vi "PPMSDR - lockin_Vsg_multichannel.vi"(6 "Vmax (end)":dbl=0.00436 format="%#_3p", 8 "Vmin (start)":dbl=-0.00364 format="%#_3p", 9 "Channels: AO":T1={"AO amp (V)"=[0.0001, 0.0, 0.0, 0.0], "AO DC (V)"=[0.00031, -0.00376, 0.0, 0.004], "AO f (Hz)"=[9.468, 0.0, 0.0, 0.0], "AO phi (deg)"=[0.0, 0.0, 0.0, 0.0], "function"=[enum."Sine Wave", enum."Sine Wave", enum."Sine Wave", enum."Sine Wave"]} {"AO DC (V)" format="%#_6p"; "AO amp (V)" format="%#_6p"}, 10 "Comments":string="DC sweep from -3.69mV to 4.31mV, 5uV step\nDragPotential sweep from -4mV to 4mV, 400uV step\nB = 0T\nT = 218mK\nVbg = 0V\nTC = 0.1s\n\nI+/-: 2/5 100uVac + DC sweep, 9.468Hz\nI2+: 28  0Vac + value according to dragpotential sweep(offset 240uV), 0Hz\nI2-: 3 0Vac + DragPotential sweep, 0Hz\nV+/-: 1/4\nV2+/-: 28/27\nV3+/-: 28/3\nappliedPotential= 0.004000", 11 "ITX folder":string="15-DragPotentialsweep-I-LDr25-RGND-Lockin") -> ()   [LabVIEW 2013]
uses:
  <userlib>/Levylab/PPMS VI/SubVI/ITX_Global.vi
  QDServer/QDServGlobal.vi
  Labview_Local/Lockin-4461_Multiple Inputs and Outputs_KH Folder/P/users1/Joe/Lockin-4461_3.0 4461-4462 Multichannel Folder/DAQ-Lockin-SubVI/Lock-in Globles Multiple Inputs and Outputs.vi
  cryogenic ltd/state machine/state machine/Cryogeni Global 1.vi
panel:
  in  "dV 2":dbl=0.0002 format="%#_3p"
  in  "Vend":dbl=-5.0 format="%#_3p"
  in  "Vstart":dbl=-4.8 format="%#_3p"
  in  "Tab Control":enum32{"Sweep BG", "lockin/SG Control", "Data"}(tab)=enum."lockin/SG Control"
  in  "dV":dbl=5e-06 format="%#_3p"
  out "T (mK)":dbl=0.24
  in  "wait between Vsgs":u32=50
  in  "Initial wait":u32=6000
  in  "# of lockins * #freq":i32=10
  in  "\"channel\" side gate":i32
  in  "T=sg\nF=bg":bool=TRUE
  in  "cycles (1,2,...)":i32=1 min=1 step=1
  in  "phase":dbl
  out "ramp rate":dbl=0.0214 format="%#_13g"
  out "Field":dbl=0.051 format="%#_13g"
  in  "function (ramp)":enum16{"Ramp", "Triangle", "Sine"}(ring)
  in  "Expt?":bool=TRUE
  out "Waveform Graph":dbl[](graph)=[-0.0036900000000000006, -0.0036850000000000008, -0.0036800000000000005, -0.0036750000000000007, -0.0036700000000000005, -0.0036650000000000007, -0.0036600000000000005, -0.0036550000000000007, -0.0036500000000000005, -0.0036450000000000007, -0.0036400000000000004, -0.0036350000000000006, -0.0036300000000000004, -0.0036250000000000006, -0.0036200000000000004, -0.0036150000000000006, -0.0036100000000000004, -0.0036050000000000006, -0.0036000000000000008, -0.0035950000000000005, -0.0035900000000000007, -0.0035850000000000005, -0.0035800000000000007, -0.0035750000000000005, -0.0035700000000000007, -0.0035650000000000005, -0.0035600000000000007, -0.0035550000000000004, -0.0035500000000000006, -0.0035450000000000004, -0.0035400000000000006, -0.0035350000000000004, -0.0035300000000000006, -0.0035250000000000004, -0.0035200000000000006, -0.0035150000000000008, -0.0035100000000000005, -0.0035050000000000007, -0.0035000000000000005, -0.0034950000000000007, -0.0034900000000000005, -0.0034850000000000007, -0.0034800000000000005, -0.0034750000000000007, -0.0034700000000000004, -0.0034650000000000006, -0.0034600000000000004, -0.0034550000000000006, -0.0034500000000000004, -0.0034450000000000006, -0.0034400000000000003, -0.0034350000000000006, -0.0034300000000000008, -0.0034250000000000005, -0.0034200000000000007, -0.0034150000000000005, -0.0034100000000000007, -0.0034050000000000005, -0.0034000000000000007, -0.0033950000000000004, -0.0033900000000000007, -0.0033850000000000004, -0.0033800000000000006, -0.0033750000000000004, -0.0033700000000000006, -0.0033650000000000004, -0.0033600000000000006, -0.0033550000000000003, -0.0033500000000000005, -0.0033450000000000008, -0.0033400000000000005, -0.0033350000000000007, -0.0033300000000000005, -0.0033250000000000007, -0.0033200000000000005, -0.0033150000000000007, -0.0033100000000000004, -0.0033050000000000006, -0.0033000000000000004, -0.0032950000000000006, -0.0032900000000000004, -0.0032850000000000006, -0.0032800000000000004, -0.0032750000000000006, -0.0032700000000000003, -0.0032650000000000005, -0.0032600000000000007, -0.0032550000000000005, -0.0032500000000000007, -0.0032450000000000005, -0.0032400000000000007, -0.0032350000000000005, -0.0032300000000000007, -0.0032250000000000004, -0.0032200000000000006, -0.0032150000000000004, -0.0032100000000000006, -0.0032050000000000004, -0.0032000000000000006, -0.003195000000000001, -0.0031900000000000006, -0.0031850000000000003, -0.0031800000000000005, -0.0031750000000000007, -0.0031700000000000005, -0.0031650000000000003, -0.0031600000000000005, -0.0031550000000000007, -0.0031500000000000005, -0.0031450000000000007, -0.0031400000000000004, -0.0031350000000000006, -0.0031300000000000004, -0.0031250000000000006, -0.0031200000000000004, -0.0031150000000000006, -0.003110000000000001, -0.0031050000000000006, -0.0031000000000000003, -0.0030950000000000005, -0.0030900000000000007, -0.0030850000000000005, -0.0030800000000000003, -0.0030750000000000005, -0.0030700000000000007, -0.0030650000000000004, -0.0030600000000000007, -0.0030550000000000004, -0.0030500000000000006, -0.0030450000000000004, -0.0030400000000000006, -0.0030350000000000004, -0.0030300000000000006, -0.0030250000000000008, -0.0030200000000000005, -0.0030150000000000003, -0.0030100000000000005, -0.0030050000000000007, -0.0030000000000000005, -0.0029950000000000003, -0.0029900000000000005, -0.0029850000000000007, -0.0029800000000000004, -0.0029750000000000006, -0.0029700000000000004, -0.0029650000000000006, -0.0029600000000000004, -0.0029550000000000006, -0.0029500000000000004, -0.0029450000000000006, -0.0029400000000000008, -0.0029350000000000005, -0.0029300000000000003, -0.0029250000000000005, -0.0029200000000000007, -0.0029150000000000005, -0.0029100000000000003, -0.0029050000000000005, -0.0029000000000000007, -0.0028950000000000004, -0.0028900000000000006, -0.0028850000000000004, -0.0028800000000000006, -0.0028750000000000004, -0.0028700000000000006, -0.0028650000000000004, -0.0028600000000000006, -0.0028550000000000008, -0.0028500000000000005, -0.0028450000000000003, -0.0028400000000000005, -0.0028350000000000007, -0.0028300000000000005, -0.0028250000000000003, -0.0028200000000000005, -0.0028150000000000007, -0.0028100000000000004, -0.0028050000000000006, -0.0028000000000000004, -0.0027950000000000006, -0.0027900000000000004, -0.0027850000000000006, -0.0027800000000000004, -0.0027750000000000006, -0.0027700000000000008, -0.0027650000000000005, -0.0027600000000000003, -0.0027550000000000005, -0.0027500000000000007, -0.0027450000000000005, -0.0027400000000000002, -0.0027350000000000005, -0.0027300000000000007, -0.0027250000000000004, -0.0027200000000000006, -0.0027150000000000004, -0.0027100000000000006, -0.002705000000000001, -0.0027000000000000006, -0.0026950000000000003, -0.0026900000000000006, -0.0026850000000000008, -0.0026800000000000005, -0.0026750000000000003, -0.0026700000000000005, -0.0026650000000000007, -0.0026600000000000005, -0.0026550000000000002, -0.0026500000000000004, -0.0026450000000000006, -0.0026400000000000004, -0.002635, -0.0026300000000000004, -0.0026250000000000006, -0.002620000000000001, -0.0026150000000000006, -0.0026100000000000003, -0.0026050000000000005, -0.0026000000000000007, -0.0025950000000000005, -0.0025900000000000003, -0.0025850000000000005, -0.0025800000000000007, -0.0025750000000000005, -0.0025700000000000002, -0.0025650000000000004, -0.0025600000000000006, -0.0025550000000000004, -0.00255, -0.0025450000000000004, -0.0025400000000000006, -0.002535000000000001, -0.0025300000000000006, -0.0025250000000000003, -0.0025200000000000005, -0.0025150000000000007, -0.0025100000000000005, -0.0025050000000000003, -0.0025000000000000005, -0.0024950000000000007, -0.0024900000000000005, -0.0024850000000000002, -0.0024800000000000004, -0.0024750000000000006, -0.0024700000000000004, -0.002465, -0.0024600000000000004, -0.0024550000000000006, -0.002450000000000001, -0.0024450000000000006, -0.0024400000000000003, -0.0024350000000000005, -0.0024300000000000007, -0.0024250000000000005, -0.0024200000000000003, -0.0024150000000000005, -0.0024100000000000007, -0.0024050000000000005, -0.0024000000000000002, -0.0023950000000000004, -0.0023900000000000006, -0.0023850000000000004, -0.00238, -0.0023750000000000004, -0.0023700000000000006, -0.0023650000000000008, -0.0023600000000000006, -0.0023550000000000003, -0.0023500000000000005, -0.0023450000000000007, -0.0023400000000000005, -0.0023350000000000003, -0.0023300000000000005, -0.0023250000000000007, -0.0023200000000000004, -0.0023150000000000002, -0.0023100000000000004, -0.0023050000000000006, -0.0023000000000000004, -0.002295, -0.0022900000000000004, -0.0022850000000000006, -0.0022800000000000008, -0.0022750000000000005, -0.0022700000000000003, -0.0022650000000000005, -0.0022600000000000007, -0.0022550000000000005, -0.0022500000000000003, -0.0022450000000000005, -0.0022400000000000007, -0.0022350000000000004, -0.00223, -0.0022250000000000004, -0.0022200000000000006, -0.0022150000000000004, -0.00221, -0.0022050000000000004, -0.0022000000000000006, -0.0021950000000000008, -0.0021900000000000005, -0.0021850000000000003, -0.0021800000000000005, -0.0021750000000000007, -0.0021700000000000005, -0.0021650000000000003, -0.0021600000000000005, -0.0021550000000000007, -0.0021500000000000004, -0.002145, -0.0021400000000000004, -0.0021350000000000006, -0.0021300000000000004, -0.002125, -0.0021200000000000004, -0.0021150000000000006, -0.0021100000000000008, -0.0021050000000000005, -0.0021000000000000003, -0.0020950000000000005, -0.0020900000000000007, -0.0020850000000000005, -0.0020800000000000003, -0.0020750000000000005, -0.0020700000000000007, -0.0020650000000000004, -0.00206, -0.0020550000000000004, -0.0020500000000000006, -0.0020450000000000004, -0.00204, -0.0020350000000000004, -0.0020300000000000006, -0.0020250000000000008, -0.0020200000000000005, -0.0020150000000000003, -0.0020100000000000005, -0.0020050000000000007, -0.0020000000000000005, -0.0019950000000000002, -0.0019900000000000004, -0.0019850000000000007, -0.0019800000000000004, -0.001975, -0.0019700000000000004, -0.0019650000000000006, -0.0019600000000000004, -0.001955, -0.0019500000000000003, -0.0019450000000000003, -0.0019400000000000005, -0.0019350000000000005, -0.0019300000000000005, -0.0019250000000000005, -0.0019200000000000005, -0.0019150000000000005, -0.0019100000000000005, -0.0019050000000000004, -0.0019000000000000004, -0.0018950000000000004, -0.0018900000000000004, -0.0018850000000000004, -0.0018800000000000004, -0.0018750000000000004, -0.0018700000000000004, -0.0018650000000000003, -0.0018600000000000003, -0.0018550000000000005, -0.0018500000000000005, -0.0018450000000000005, -0.0018400000000000005, -0.0018350000000000005, -0.0018300000000000005, -0.0018250000000000004, -0.0018200000000000004, -0.0018150000000000004, -0.0018100000000000004, -0.0018050000000000004, -0.0018000000000000004, -0.0017950000000000004, -0.0017900000000000004, -0.0017850000000000003, -0.0017800000000000003, -0.0017750000000000003, -0.0017700000000000003, -0.0017650000000000005, -0.0017600000000000005, -0.0017550000000000005, -0.0017500000000000005, -0.0017450000000000005, -0.0017400000000000004, -0.0017350000000000004, -0.0017300000000000002, -0.0017250000000000004, -0.0017200000000000006, -0.0017150000000000004, -0.0017100000000000006, -0.0017050000000000004, -0.0017000000000000006, -0.0016950000000000003, -0.0016900000000000005, -0.0016850000000000003, -0.0016800000000000005, -0.0016750000000000003, -0.0016700000000000005, -0.0016650000000000002, -0.0016600000000000005, -0.0016550000000000002, -0.0016500000000000004, -0.0016450000000000002, -0.0016400000000000004, -0.0016350000000000006, -0.0016300000000000004, -0.0016250000000000006, -0.0016200000000000003, -0.0016150000000000005, -0.0016100000000000003, -0.0016050000000000005, -0.0016000000000000003, -0.0015950000000000005, -0.0015900000000000003, -0.0015850000000000005, -0.0015800000000000002, -0.0015750000000000004, -0.0015700000000000002, -0.0015650000000000004, -0.0015600000000000002, -0.0015550000000000004, -0.0015500000000000006, -0.0015450000000000004, -0.0015400000000000006, -0.0015350000000000003, -0.0015300000000000005, -0.0015250000000000003, -0.0015200000000000005, -0.0015150000000000003, -0.0015100000000000005, -0.0015050000000000003, -0.0015000000000000005, -0.0014950000000000002, -0.0014900000000000004, -0.0014850000000000002, -0.0014800000000000004, -0.0014750000000000002, -0.0014700000000000004, -0.0014650000000000006, -0.0014600000000000004, -0.0014550000000000006, -0.0014500000000000003, -0.0014450000000000005, -0.0014400000000000003, -0.0014350000000000005, -0.0014300000000000003, -0.0014250000000000005, -0.0014200000000000003, -0.0014150000000000005, -0.0014100000000000002, -0.0014050000000000004, -0.0014000000000000002, -0.0013950000000000004, -0.0013900000000000002, -0.0013850000000000004, -0.0013800000000000006, -0.0013750000000000004, -0.0013700000000000006, -0.0013650000000000003, -0.0013600000000000005, -0.0013550000000000003, -0.0013500000000000005, -0.0013450000000000003, -0.0013400000000000005, -0.0013350000000000002, -0.0013300000000000005, -0.0013250000000000002, -0.0013200000000000004, -0.0013150000000000002, -0.0013100000000000004, -0.0013050000000000002, -0.0013000000000000004, -0.0012950000000000006, -0.0012900000000000003, -0.0012850000000000006, -0.0012800000000000003, -0.0012750000000000005, -0.0012700000000000003, -0.0012650000000000005, -0.0012600000000000003, -0.0012550000000000005, -0.0012500000000000002, -0.0012450000000000004, -0.0012400000000000002, -0.0012350000000000004, -0.0012300000000000002, -0.0012250000000000004, -0.0012200000000000002, -0.0012150000000000004, -0.0012100000000000006, -0.0012050000000000003, -0.0012000000000000005, -0.0011950000000000003, -0.0011900000000000005, -0.0011850000000000003, -0.0011800000000000005, -0.0011750000000000003, -0.0011700000000000005, -0.0011650000000000002, -0.0011600000000000004, -0.0011550000000000002, -0.0011500000000000004, -0.0011450000000000002, -0.0011400000000000004, -0.0011350000000000002, -0.0011300000000000004, -0.0011250000000000006, -0.0011200000000000003, -0.0011150000000000005, -0.0011100000000000003, -0.0011050000000000005, -0.0011000000000000003, -0.0010950000000000005, -0.0010900000000000003, -0.0010850000000000005, -0.0010800000000000002, -0.0010750000000000004, -0.0010700000000000002, -0.0010650000000000004, -0.0010600000000000002, -0.0010550000000000004, -0.0010500000000000002, -0.0010450000000000004, -0.0010400000000000006, -0.0010350000000000003, -0.0010300000000000005, -0.0010250000000000003, -0.0010200000000000005, -0.0010150000000000003, -0.0010100000000000005, -0.0010050000000000003, -0.0010000000000000005, -0.0009950000000000002, -0.0009900000000000004, -0.0009850000000000002, -0.0009800000000000004, -0.0009750000000000002, -0.0009700000000000004, -0.0009650000000000001, -0.0009600000000000003, -0.0009550000000000006, -0.0009500000000000003, -0.0009450000000000005, -0.0009400000000000003, -0.0009350000000000005, -0.0009300000000000003, -0.0009250000000000005, -0.0009200000000000002, -0.0009150000000000004, -0.0009100000000000002, -0.0009050000000000004, -0.0009000000000000002, -0.0008950000000000004, -0.0008900000000000002, -0.0008850000000000004, -0.0008800000000000001, -0.0008750000000000003, -0.0008700000000000005, -0.0008650000000000003, -0.0008600000000000005, -0.0008550000000000003, -0.0008500000000000005, -0.0008450000000000003, -0.0008400000000000005, -0.0008350000000000002, -0.0008300000000000004, -0.0008250000000000002, -0.0008200000000000004, -0.0008150000000000002, -0.0008100000000000004, -0.0008050000000000002, -0.0008000000000000004, -0.0007950000000000001, -0.0007900000000000003, -0.0007850000000000005, -0.0007800000000000003, -0.0007750000000000005, -0.0007700000000000003, -0.0007650000000000005, -0.0007600000000000003, -0.0007550000000000005, -0.0007500000000000002, -0.0007450000000000004, -0.0007400000000000002, -0.0007350000000000004, -0.0007300000000000002, -0.0007250000000000004, -0.0007200000000000002, -0.0007150000000000004, -0.0007100000000000001, -0.0007050000000000003, -0.0007000000000000005, -0.0006950000000000003, -0.0006900000000000005, -0.0006850000000000003, -0.0006800000000000005, -0.0006750000000000003, -0.0006700000000000005, -0.0006650000000000002, -0.0006600000000000004, -0.0006550000000000002, -0.0006500000000000004, -0.0006450000000000002, -0.0006400000000000004, -0.0006350000000000001, -0.0006300000000000004, -0.0006250000000000001, -0.0006200000000000003, -0.0006150000000000005, -0.0006100000000000003, -0.0006050000000000005, -0.0006000000000000003, -0.0005950000000000005, -0.0005900000000000002, -0.0005850000000000005, -0.0005800000000000002, -0.0005750000000000004, -0.0005700000000000002, -0.0005650000000000004, -0.0005600000000000002, -0.0005550000000000004, -0.0005500000000000001, -0.0005450000000000003, -0.0005400000000000001, -0.0005350000000000003, -0.0005300000000000005, -0.0005250000000000003, -0.0005200000000000005, -0.0005150000000000003, -0.0005100000000000005, -0.0005050000000000002, -0.0005000000000000004, -0.0004950000000000002, -0.0004900000000000004, -0.0004850000000000002, -0.0004800000000000004, -0.00047500000000000016, -0.00047000000000000037, -0.00046500000000000014, -0.00046000000000000034, -0.0004550000000000001, -0.0004500000000000003, -0.0004450000000000005, -0.0004400000000000003, -0.0004350000000000005, -0.00043000000000000026, -0.00042500000000000046, -0.00042000000000000023, -0.00041500000000000044, -0.0004100000000000002, -0.0004050000000000004, -0.0004000000000000002, -0.0003950000000000004, -0.00039000000000000016, -0.00038500000000000036, -0.00038000000000000013, -0.00037500000000000033, -0.0003700000000000001, -0.0003650000000000003, -0.0003600000000000005, -0.0003550000000000003, -0.0003500000000000005, -0.00034500000000000025, -0.00034000000000000046, -0.00033500000000000023, -0.00033000000000000043, -0.0003250000000000002, -0.0003200000000000004, -0.0003150000000000002, -0.0003100000000000004, -0.00030500000000000015, -0.00030000000000000035, -0.0002950000000000001, -0.0002900000000000003, -0.0002850000000000001, -0.0002800000000000003, -0.0002750000000000005, -0.0002700000000000003, -0.0002650000000000005, -0.00026000000000000025, -0.00025500000000000045, -0.0002500000000000002, -0.0002450000000000004, -0.0002400000000000002, -0.0002350000000000004, -0.00023000000000000017, -0.00022500000000000037, -0.00022000000000000014, -0.00021500000000000035, -0.00021000000000000012, -0.00020500000000000032, -0.0002000000000000001, -0.0001950000000000003, -0.0001900000000000005, -0.00018500000000000027, -0.00018000000000000047, -0.00017500000000000024, -0.00017000000000000045, -0.00016500000000000022, -0.00016000000000000042, -0.0001550000000000002, -0.0001500000000000004, -0.00014500000000000016, -0.00014000000000000037, -0.00013500000000000014, -0.00013000000000000034, -0.0001250000000000001, -0.00012000000000000031, -0.00011500000000000008, -0.00011000000000000029, -0.00010500000000000049, -0.00010000000000000026, -9.500000000000047e-05, -9.000000000000024e-05, -8.500000000000044e-05, -8.000000000000021e-05, -7.500000000000041e-05, -7.000000000000018e-05, -6.500000000000039e-05, -6.000000000000016e-05, -5.500000000000036e-05, -5.000000000000013e-05, -4.5000000000000335e-05, -4.0000000000000105e-05, -3.500000000000031e-05, -3.000000000000008e-05, -2.5000000000000282e-05, -2.0000000000000486e-05, -1.5000000000000256e-05, -1.000000000000046e-05, -5.00000000000023e-06, -4.336808689942018e-19, 4.999999999999796e-06, 9.999999999999593e-06, 1.4999999999999823e-05, 1.999999999999962e-05, 2.499999999999985e-05, 2.9999999999999645e-05, 3.4999999999999875e-05, 3.999999999999967e-05, 4.49999999999999e-05, 4.99999999999997e-05, 5.499999999999993e-05, 5.9999999999999724e-05, 6.499999999999952e-05, 6.999999999999975e-05, 7.499999999999955e-05, 7.999999999999978e-05, 8.499999999999957e-05, 8.99999999999998e-05, 9.49999999999996e-05, 9.999999999999983e-05, 0.00010499999999999962, 0.00010999999999999985, 0.00011499999999999965, 0.00011999999999999988, 0.00012499999999999968, 0.0001299999999999999, 0.0001349999999999997, 0.00013999999999999993, 0.00014499999999999973, 0.00014999999999999996, 0.00015499999999999976, 0.00015999999999999955, 0.00016499999999999978, 0.00016999999999999958, 0.0001749999999999998, 0.0001799999999999996, 0.00018499999999999983, 0.00018999999999999963, 0.00019499999999999986, 0.00019999999999999966, 0.0002049999999999999, 0.00020999999999999968, 0.0002149999999999999, 0.0002199999999999997, 0.0002249999999999995, 0.00023000000000000017, 0.00023499999999999997, 0.00023999999999999976, 0.00024499999999999956, 0.00024999999999999935, 0.000255, 0.0002599999999999998, 0.0002649999999999996, 0.0002699999999999994, 0.00027500000000000007, 0.00027999999999999987, 0.00028499999999999966, 0.00028999999999999946, 0.0002950000000000001, 0.0002999999999999999, 0.0003049999999999997, 0.0003099999999999995, 0.0003150000000000002, 0.00031999999999999997, 0.00032499999999999977, 0.00032999999999999956, 0.00033499999999999936, 0.00034, 0.0003449999999999998, 0.0003499999999999996, 0.0003549999999999994, 0.0003600000000000001, 0.0003649999999999999, 0.00036999999999999967, 0.00037499999999999947, 0.00038000000000000013, 0.0003849999999999999, 0.0003899999999999997, 0.0003949999999999995, 0.0004000000000000002, 0.000405, 0.0004099999999999998, 0.00041499999999999957, 0.00041999999999999937, 0.00042500000000000003, 0.0004299999999999998, 0.0004349999999999996, 0.0004399999999999994, 0.0004450000000000001, 0.0004499999999999999, 0.0004549999999999997, 0.00045999999999999947, 0.00046500000000000014, 0.00046999999999999993, 0.00047499999999999973, 0.0004799999999999995, 0.0004850000000000002, 0.00049, 0.0004949999999999998, 0.0004999999999999996, 0.0005049999999999994, 0.00051, 0.0005149999999999998, 0.0005199999999999996, 0.0005249999999999994, 0.0005300000000000001, 0.0005349999999999999, 0.0005399999999999997, 0.0005449999999999995, 0.0005500000000000001, 0.0005549999999999999, 0.0005599999999999997, 0.0005649999999999995, 0.0005700000000000002, 0.000575, 0.0005799999999999998, 0.0005849999999999996, 0.0005899999999999994, 0.000595, 0.0005999999999999998, 0.0006049999999999996, 0.0006099999999999994, 0.0006150000000000001, 0.0006199999999999999, 0.0006249999999999997, 0.0006299999999999995, 0.0006350000000000001, 0.0006399999999999999, 0.0006449999999999997, 0.0006499999999999995, 0.0006550000000000002, 0.00066, 0.0006649999999999998, 0.0006699999999999996, 0.0006749999999999994, 0.00068, 0.0006849999999999998, 0.0006899999999999996, 0.0006949999999999994, 0.0007000000000000001, 0.0007049999999999999, 0.0007099999999999997, 0.0007149999999999995, 0.0007200000000000002, 0.000725, 0.0007299999999999997, 0.0007349999999999995, 0.0007400000000000002, 0.000745, 0.0007499999999999998, 0.0007549999999999996, 0.0007599999999999994, 0.0007650000000000001, 0.0007699999999999999, 0.0007749999999999996, 0.0007799999999999994, 0.0007850000000000001, 0.0007899999999999999, 0.0007949999999999997, 0.0007999999999999995, 0.0008050000000000002, 0.00081, 0.0008149999999999998, 0.0008199999999999995, 0.0008250000000000002, 0.00083, 0.0008349999999999998, 0.0008399999999999996, 0.0008449999999999994, 0.0008500000000000001, 0.0008549999999999999, 0.0008599999999999997, 0.0008649999999999994, 0.0008700000000000001, 0.0008749999999999999, 0.0008799999999999997, 0.0008849999999999995, 0.0008900000000000002, 0.000895, 0.0008999999999999998, 0.0009049999999999996, 0.0009100000000000002, 0.000915, 0.0009199999999999998, 0.0009249999999999996, 0.0009299999999999994, 0.0009350000000000001, 0.0009399999999999999, 0.0009449999999999997, 0.0009499999999999995, 0.0009550000000000001, 0.0009599999999999999, 0.0009649999999999997, 0.0009699999999999995, 0.0009750000000000002, 0.00098, 0.0009849999999999998, 0.0009899999999999996, 0.0009950000000000002, 0.001, 0.0010049999999999998, 0.0010099999999999996, 0.0010149999999999994, 0.00102, 0.0010249999999999999, 0.0010299999999999997, 0.0010349999999999995, 0.0010400000000000001, 0.001045, 0.0010499999999999997, 0.0010549999999999995, 0.0010600000000000002, 0.001065, 0.0010699999999999998, 0.0010749999999999996, 0.0010800000000000002, 0.001085, 0.0010899999999999998, 0.0010949999999999996, 0.0010999999999999994, 0.001105, 0.0011099999999999999, 0.0011149999999999997, 0.0011199999999999995, 0.0011250000000000001, 0.00113, 0.0011349999999999997, 0.0011399999999999995, 0.0011450000000000002, 0.00115, 0.0011549999999999998, 0.0011599999999999996, 0.0011650000000000002, 0.00117, 0.0011749999999999998, 0.0011799999999999996, 0.0011849999999999994, 0.00119, 0.0011949999999999999, 0.0011999999999999997, 0.0012049999999999995, 0.0012100000000000001, 0.001215, 0.0012199999999999997, 0.0012249999999999995, 0.0012300000000000002, 0.001235, 0.0012399999999999998, 0.0012449999999999996, 0.0012500000000000002, 0.001255, 0.0012599999999999998, 0.0012649999999999996, 0.0012699999999999994, 0.001275, 0.0012799999999999999, 0.0012849999999999997, 0.0012899999999999995, 0.0012950000000000001, 0.0013, 0.0013049999999999997, 0.0013099999999999995, 0.0013150000000000002, 0.00132, 0.0013249999999999998, 0.0013299999999999996, 0.0013350000000000002, 0.00134, 0.0013449999999999998, 0.0013499999999999996, 0.0013549999999999994, 0.00136, 0.001365, 0.0013699999999999997, 0.0013749999999999995, 0.0013800000000000002, 0.001385, 0.0013899999999999997, 0.0013949999999999995, 0.0014000000000000002, 0.001405, 0.0014099999999999998, 0.0014149999999999996, 0.0014200000000000003, 0.001425, 0.0014299999999999998, 0.0014349999999999996, 0.0014399999999999994, 0.001445, 0.00145, 0.0014549999999999997, 0.0014599999999999995, 0.0014650000000000002, 0.00147, 0.0014749999999999997, 0.0014799999999999995, 0.0014850000000000002, 0.00149, 0.0014949999999999998, 0.0014999999999999996, 0.0015050000000000003, 0.00151, 0.0015149999999999999, 0.0015199999999999997, 0.0015249999999999994, 0.0015300000000000001, 0.001535, 0.0015399999999999997, 0.0015449999999999995, 0.0015500000000000002, 0.001555, 0.0015599999999999998, 0.0015649999999999996, 0.0015700000000000002, 0.001575, 0.0015799999999999998, 0.0015849999999999996, 0.0015900000000000003, 0.001595, 0.0015999999999999999, 0.0016049999999999997, 0.0016099999999999995, 0.0016150000000000001, 0.00162, 0.0016249999999999997, 0.0016299999999999995, 0.0016350000000000002, 0.00164, 0.0016449999999999998, 0.0016499999999999996, 0.0016550000000000002, 0.00166, 0.0016649999999999998, 0.0016699999999999996, 0.0016750000000000003, 0.00168, 0.0016849999999999999, 0.0016899999999999997, 0.0016949999999999995, 0.0017000000000000001, 0.001705, 0.0017099999999999997, 0.0017149999999999995, 0.0017200000000000002, 0.001725, 0.0017299999999999998, 0.0017349999999999996, 0.0017400000000000002, 0.001745, 0.0017499999999999998, 0.0017549999999999996, 0.0017600000000000003, 0.001765, 0.0017699999999999999, 0.0017749999999999997, 0.0017799999999999995, 0.0017850000000000001, 0.00179, 0.0017949999999999997, 0.0017999999999999995, 0.0018050000000000002, 0.00181, 0.0018149999999999998, 0.0018199999999999996, 0.0018250000000000002, 0.00183, 0.0018349999999999998, 0.0018399999999999996, 0.0018450000000000003, 0.00185, 0.0018549999999999999, 0.0018599999999999997, 0.0018649999999999995, 0.0018700000000000001, 0.001875, 0.0018799999999999997, 0.0018849999999999995, 0.0018900000000000002, 0.001895, 0.0018999999999999998, 0.0019049999999999996, 0.0019100000000000002, 0.001915, 0.0019199999999999998, 0.0019249999999999996, 0.0019300000000000003, 0.001935, 0.0019399999999999999, 0.0019449999999999997, 0.0019499999999999995, 0.001955, 0.00196, 0.0019649999999999997, 0.0019699999999999995, 0.001975, 0.00198, 0.001985, 0.0019899999999999996, 0.0019950000000000002, 0.002, 0.002005, 0.0020099999999999996, 0.0020150000000000003, 0.00202, 0.002025, 0.0020299999999999997, 0.0020349999999999995, 0.00204, 0.002045, 0.0020499999999999997, 0.0020549999999999995, 0.00206, 0.002065, 0.00207, 0.0020749999999999996, 0.0020800000000000003, 0.002085, 0.00209, 0.0020949999999999996, 0.0021000000000000003, 0.002105, 0.00211, 0.0021149999999999997, 0.0021199999999999995, 0.002125, 0.00213, 0.0021349999999999997, 0.0021399999999999995, 0.002145, 0.00215, 0.002155, 0.0021599999999999996, 0.0021650000000000003, 0.00217, 0.002175, 0.0021799999999999996, 0.0021850000000000003, 0.00219, 0.002195, 0.0021999999999999997, 0.0022049999999999995, 0.00221, 0.002215, 0.0022199999999999998, 0.0022249999999999995, 0.00223, 0.002235, 0.00224, 0.0022449999999999996, 0.0022500000000000003, 0.002255, 0.00226, 0.0022649999999999997, 0.0022700000000000003, 0.002275, 0.00228, 0.0022849999999999997, 0.0022899999999999995, 0.002295, 0.0023, 0.0023049999999999998, 0.0023099999999999996, 0.0023150000000000002, 0.00232, 0.002325, 0.0023299999999999996, 0.0023350000000000003, 0.00234, 0.002345, 0.0023499999999999997, 0.0023550000000000003, 0.00236, 0.002365, 0.0023699999999999997, 0.0023749999999999995, 0.00238, 0.002385, 0.0023899999999999998, 0.0023949999999999996, 0.0024000000000000002, 0.002405, 0.00241, 0.0024149999999999996, 0.0024200000000000003, 0.002425, 0.00243, 0.0024349999999999997, 0.0024400000000000003, 0.002445, 0.00245, 0.0024549999999999997, 0.0024599999999999995, 0.002465, 0.00247, 0.0024749999999999998, 0.0024799999999999996, 0.0024850000000000002, 0.00249, 0.002495, 0.0024999999999999996, 0.0025050000000000003, 0.00251, 0.002515, 0.0025199999999999997, 0.0025250000000000003, 0.00253, 0.002535, 0.0025399999999999997, 0.0025449999999999995, 0.00255, 0.002555, 0.0025599999999999998, 0.0025649999999999996, 0.0025700000000000002, 0.002575, 0.00258, 0.0025849999999999996, 0.0025900000000000003, 0.002595, 0.0026, 0.0026049999999999997, 0.0026100000000000003, 0.002615, 0.00262, 0.0026249999999999997, 0.0026299999999999995, 0.002635, 0.00264, 0.0026449999999999998, 0.0026499999999999996, 0.0026550000000000002, 0.00266, 0.002665, 0.0026699999999999996, 0.0026750000000000003, 0.00268, 0.002685, 0.0026899999999999997, 0.0026950000000000003, 0.0027, 0.002705, 0.0027099999999999997, 0.0027149999999999995, 0.00272, 0.002725, 0.00273, 0.0027349999999999996, 0.0027400000000000002, 0.002745, 0.00275, 0.0027549999999999996, 0.0027600000000000003, 0.002765, 0.00277, 0.0027749999999999997, 0.0027800000000000004, 0.002785, 0.00279, 0.0027949999999999997, 0.0027999999999999995, 0.002805, 0.00281, 0.002815, 0.0028199999999999996, 0.0028250000000000003, 0.00283, 0.002835, 0.0028399999999999996, 0.0028450000000000003, 0.00285, 0.002855, 0.0028599999999999997, 0.0028650000000000004, 0.00287, 0.002875, 0.0028799999999999997, 0.0028849999999999995, 0.00289, 0.002895, 0.0029, 0.0029049999999999996, 0.0029100000000000003, 0.002915, 0.00292, 0.0029249999999999996, 0.0029300000000000003, 0.002935, 0.00294, 0.0029449999999999997, 0.0029500000000000004, 0.002955, 0.00296, 0.0029649999999999998, 0.0029699999999999996, 0.002975, 0.00298, 0.002985, 0.0029899999999999996, 0.0029950000000000003, 0.003, 0.003005, 0.0030099999999999997, 0.0030150000000000003, 0.00302, 0.003025, 0.0030299999999999997, 0.0030350000000000004, 0.00304, 0.003045, 0.0030499999999999998, 0.0030549999999999996, 0.0030600000000000002, 0.003065, 0.00307, 0.0030749999999999996, 0.0030800000000000003, 0.003085, 0.00309, 0.0030949999999999997, 0.0031000000000000003, 0.003105, 0.00311, 0.0031149999999999997, 0.0031200000000000004, 0.003125, 0.00313, 0.0031349999999999998, 0.0031399999999999996, 0.0031450000000000002, 0.00315, 0.003155, 0.0031599999999999996, 0.0031650000000000003, 0.00317, 0.003175, 0.0031799999999999997, 0.0031850000000000003, 0.00319, 0.003195, 0.0031999999999999997, 0.0032050000000000004, 0.00321, 0.003215, 0.0032199999999999998, 0.0032249999999999996, 0.0032300000000000002, 0.003235, 0.00324, 0.0032449999999999996, 0.0032500000000000003, 0.003255, 0.00326, 0.0032649999999999997, 0.0032700000000000003, 0.003275, 0.00328, 0.0032849999999999997, 0.0032900000000000004, 0.003295, 0.0033, 0.0033049999999999998, 0.0033099999999999996, 0.0033150000000000002, 0.00332, 0.003325, 0.0033299999999999996, 0.0033350000000000003, 0.00334, 0.003345, 0.0033499999999999997, 0.0033550000000000003, 0.00336, 0.003365, 0.0033699999999999997, 0.0033750000000000004, 0.00338, 0.003385, 0.00339, 0.0033949999999999996, 0.0034000000000000002, 0.003405, 0.00341, 0.0034149999999999996, 0.0034200000000000003, 0.003425, 0.00343, 0.0034349999999999997, 0.0034400000000000003, 0.003445, 0.00345, 0.0034549999999999997, 0.0034600000000000004, 0.003465, 0.00347, 0.003475, 0.0034799999999999996, 0.0034850000000000003, 0.00349, 0.003495, 0.0034999999999999996, 0.0035050000000000003, 0.00351, 0.003515, 0.0035199999999999997, 0.0035250000000000004, 0.00353, 0.003535, 0.0035399999999999997, 0.0035450000000000004, 0.00355, 0.003555, 0.00356, 0.0035649999999999996, 0.0035700000000000003, 0.003575, 0.00358, 0.0035849999999999996, 0.0035900000000000003, 0.003595, 0.0036, 0.0036049999999999997, 0.0036100000000000004, 0.003615, 0.00362, 0.0036249999999999998, 0.0036300000000000004, 0.003635, 0.00364, 0.003645, 0.0036499999999999996, 0.0036550000000000003, 0.00366, 0.003665, 0.0036699999999999997, 0.0036750000000000003, 0.00368, 0.003685, 0.0036899999999999997, 0.0036950000000000004, 0.0037, 0.003705, 0.0037099999999999998, 0.0037150000000000004, 0.00372, 0.003725, 0.00373, 0.0037349999999999996, 0.0037400000000000003, 0.003745, 0.00375, 0.0037549999999999997, 0.0037600000000000003, 0.003765, 0.00377, 0.0037749999999999997, 0.0037800000000000004, 0.003785, 0.00379, 0.0037949999999999998, 0.0038000000000000004, 0.0038050000000000002, 0.00381, 0.003815, 0.0038199999999999996, 0.0038250000000000003, 0.00383, 0.003835, 0.0038399999999999997, 0.0038450000000000003, 0.00385, 0.003855, 0.0038599999999999997, 0.0038650000000000004, 0.00387, 0.003875, 0.0038799999999999998, 0.0038850000000000004, 0.0038900000000000002, 0.003895, 0.0039, 0.0039049999999999996, 0.00391, 0.003915, 0.00392, 0.003925, 0.00393, 0.003935, 0.00394, 0.003945, 0.00395, 0.003955, 0.00396, 0.003965, 0.0039700000000000004, 0.003975, 0.00398, 0.003985, 0.0039900000000000005, 0.003995, 0.004, 0.004005, 0.00401, 0.004015, 0.00402, 0.004025, 0.00403, 0.004035, 0.00404, 0.004045, 0.00405, 0.0040550000000000004, 0.00406, 0.004065, 0.00407, 0.0040750000000000005, 0.00408, 0.004085, 0.00409, 0.004095, 0.0041, 0.004105, 0.00411, 0.004115, 0.00412, 0.004125, 0.00413, 0.004135, 0.00414, 0.004144999999999999, 0.004150000000000001, 0.004155000000000001, 0.0041600000000000005, 0.004165, 0.00417, 0.004175, 0.00418, 0.0041849999999999995, 0.004189999999999999, 0.004195000000000001, 0.004200000000000001, 0.004205, 0.00421, 0.004215, 0.00422, 0.004225, 0.004229999999999999, 0.004235000000000001, 0.004240000000000001, 0.0042450000000000005, 0.00425, 0.004255, 0.00426, 0.004265, 0.0042699999999999995, 0.004274999999999999, 0.004280000000000001, 0.004285000000000001, 0.00429, 0.004295, 0.0043, 0.004305, 0.00431]
  out "Lockins":cluster{"Y":dbl[], "Y":dbl[]}[](graph)
  out "Lockins 2":cluster{"Y":dbl[], "Y":dbl[]}[](graph)
  out "Lockins 3":cluster{"Y":dbl[], dbl[]}[](graph)
  in  "Current channels":i32[](array[numeric])=[0, 0, 0]
  in  "Voltage channels":i32[](array[numeric])=[2, 3, 4]
  # "Vsg start = Vmin + X*B\nVsg end = Vsg start + Vmax\nMAKE X=0 IF YOU WANT TO\nSWEEP THE REGULAR WAY"
  # "0"
  # "1"
  # "2"
  # "3"
  # "4"
  # "5"
  # "6"
  # "7"
  # "V sg"
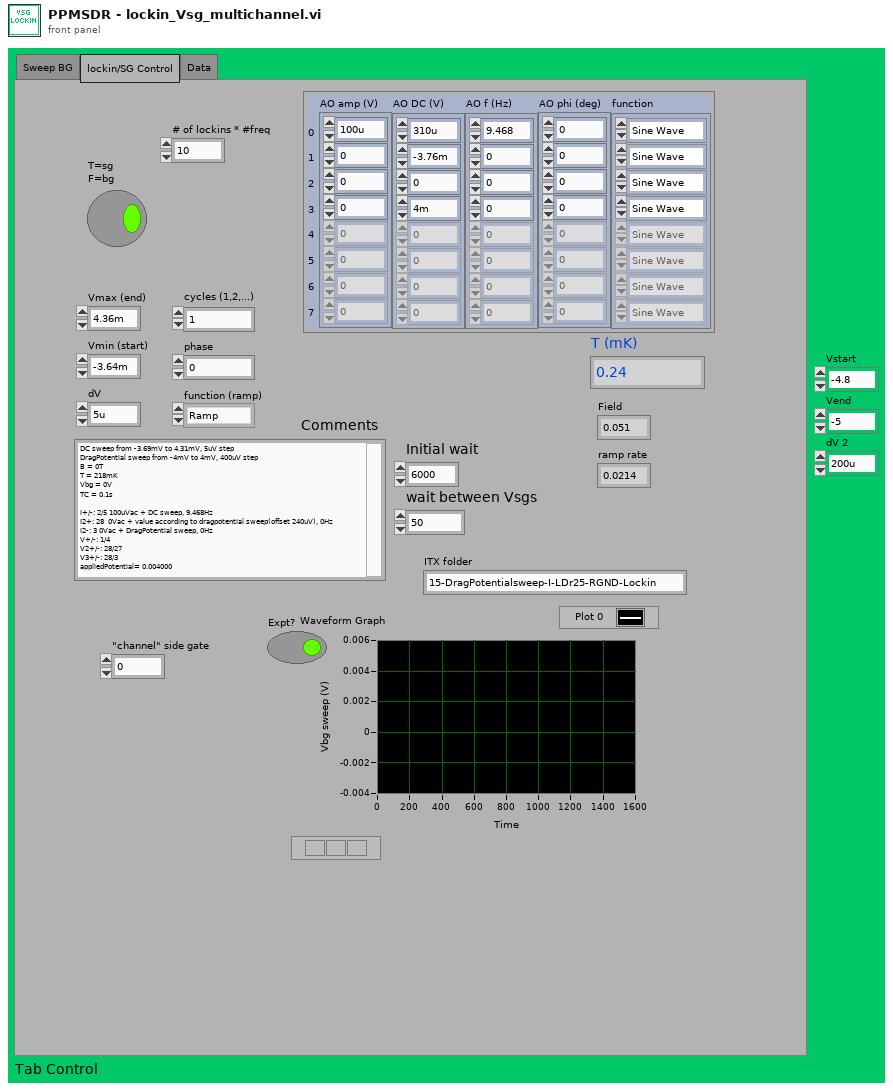
[diagram p1: front panel]
types:
  T1 = cluster{"AO amp (V)":dbl[], "AO DC (V)":dbl[], "AO f (Hz)":dbl[], "AO phi (deg)":dbl[], "function":enum16{"Sine Wave", "Triangle Wave", "Square Wave", "Sawtooth Wave"}[]}
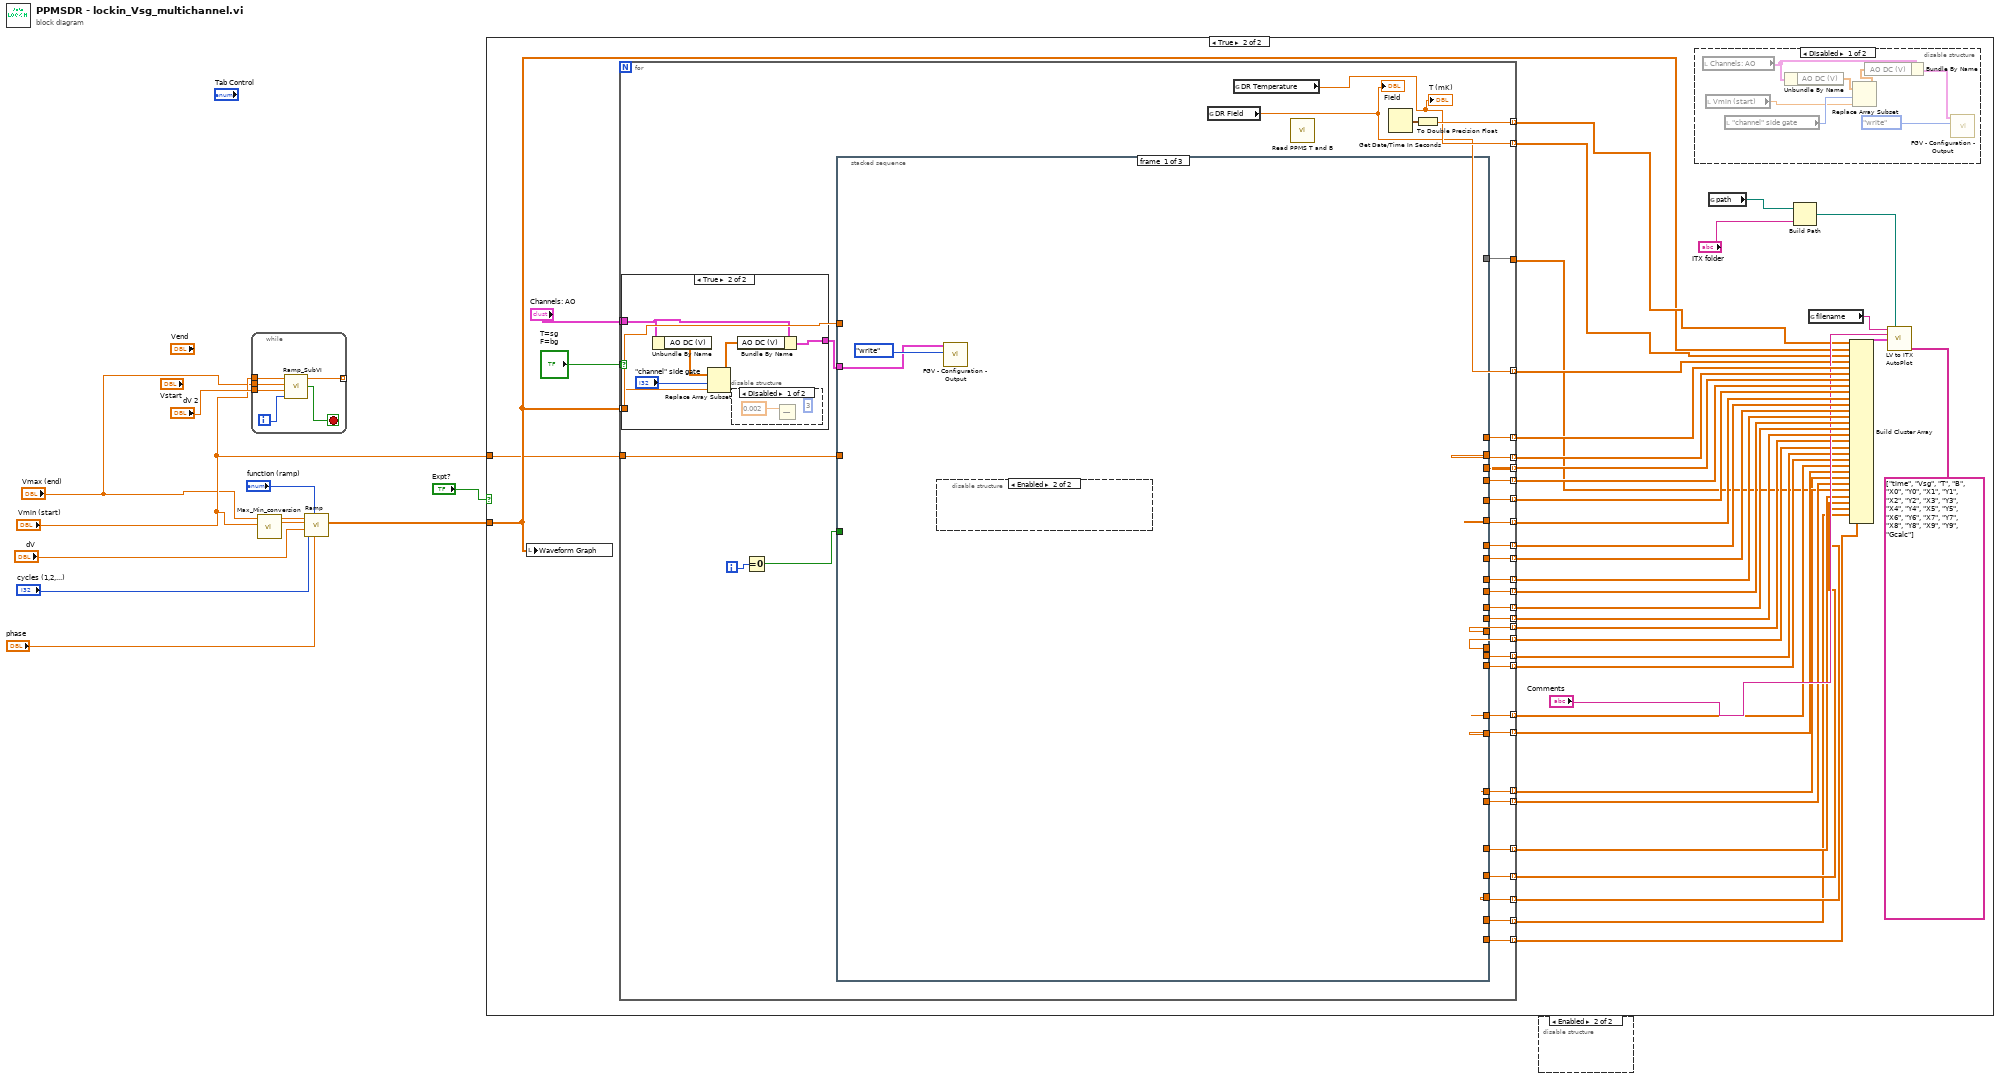
[diagram p0: block diagram]
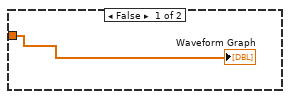
[diagram p2: hidden frame]
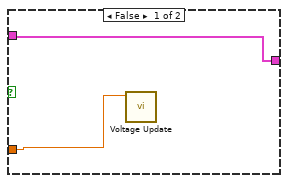
[diagram p4: hidden frame]
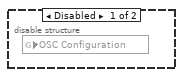
[diagram p6: hidden frame]
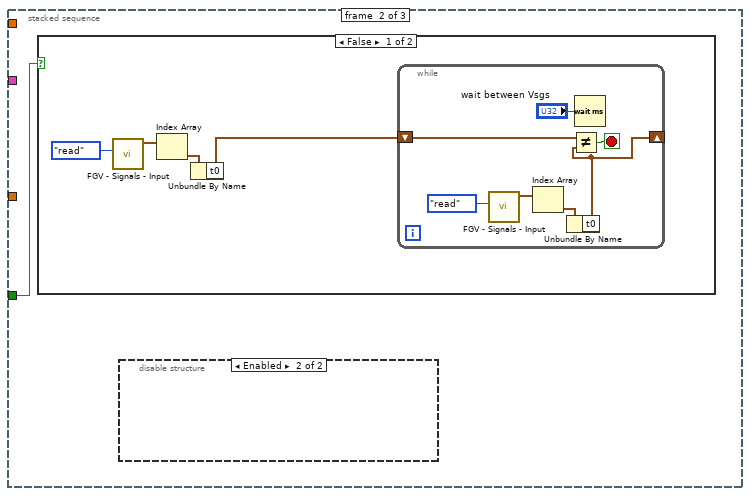
[diagram p7: hidden frame]
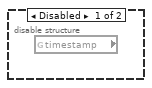
[diagram p8: hidden frame]
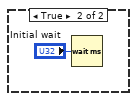
[diagram p9: hidden frame]
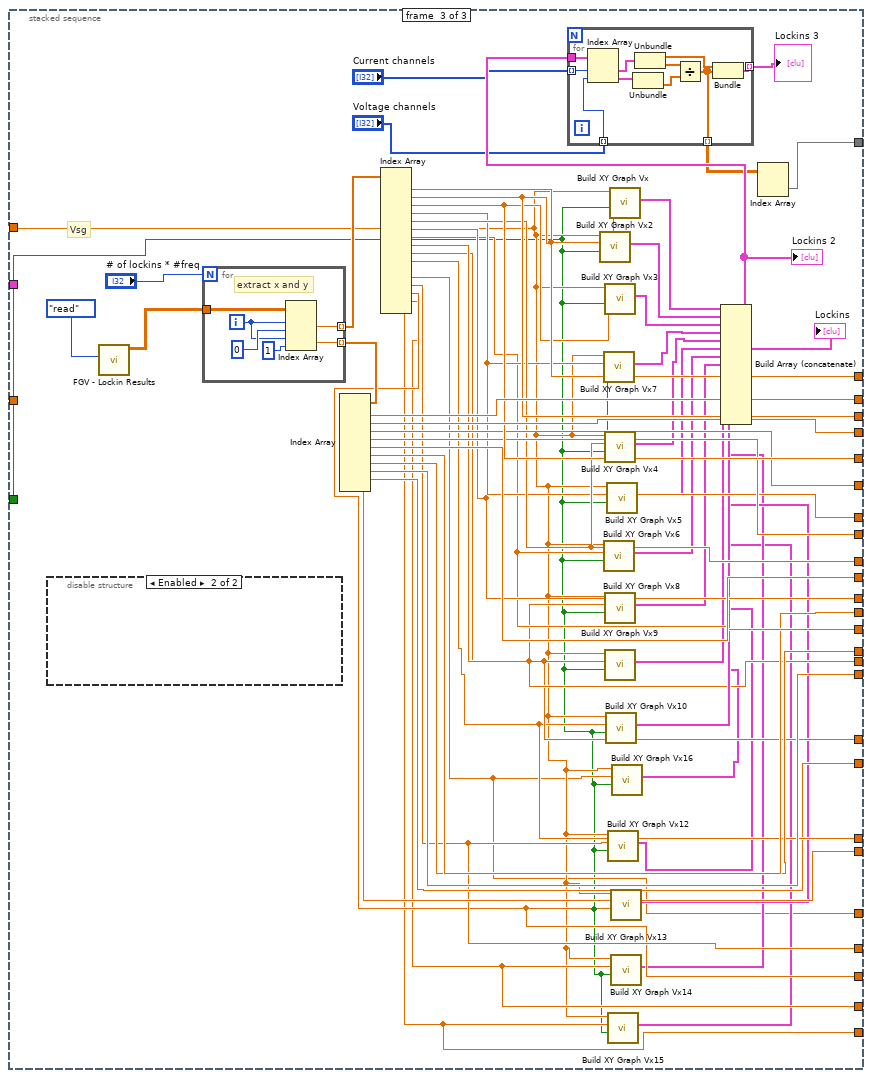
[diagram p10: hidden frame]
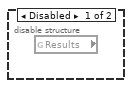
[diagram p11: hidden frame]
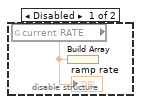
[diagram p12: hidden frame]
diagram:
  n1 = while {
    tunnel: "Vmin (start)" -> [w17]
    tunnel: "Vmax (end)" -> [w16]
    tunnel: "dV 2" -> [w15]
    tunnel: [w12] -> _ mode=indexing
    i -> [w14]
    stop <- w13 stop-if-true
    n2 = call <userlib>:"Ramp_SubVI.vi"("index"=w14, "step"=w15, "end"=w16, "start"=w17) -> ("Stop?"=w13:bool, "Numeric"=w12:dbl)  [unwired: 1 in]
  }
  n3 = call <userlib>:"Max_Min_conversion.vi"("Min"="Vmin (start)", "Max"="Vmax (end)") -> ("offset"=w10:dbl, "Amplitude"=w11:dbl)  [unwired: 8 in]
  n4 = call <userlib>:"Ramp.vi"("phase"="phase", "function (ramp)"="function (ramp)", "cycles (1,2,...)"="cycles (1,2,...)", "step size"="dV", "offset"=w10, "amplitude"=w11) -> ("Waveform Graph"=w1:dbl[])  [unwired: 3 in, 2 out]
  n5 = case shown="True" "Expt?" {
    tunnel: w1 -> [w18 w26]
    tunnel: "Vmin (start)" -> [_ w19]
    frame False {
      "Waveform Graph" <- w18
    }
    frame True {
      n6 = local write "Waveform Graph"(w26) -> ()
      n7 = for {
        tunnel: "Channels: AO" -> [w102]
        tunnel: w26 -> [w92] mode=indexing
        tunnel: [w98] -> w50 mode=indexing
        tunnel: [w97] -> w52 mode=indexing
        tunnel: [w96] -> w51 mode=indexing
        tunnel: [w95] -> w49 mode=indexing
        tunnel: [w94] -> w48 mode=indexing
        tunnel: [w93] -> w47 mode=indexing
        tunnel: [w91] -> w46 mode=indexing
        tunnel: [w90] -> w45 mode=indexing
        tunnel: [w89] -> w44 mode=indexing
        tunnel: [w88] -> w43 mode=indexing
        tunnel: [w87] -> w41 mode=indexing
        tunnel: [w86] -> w42 mode=indexing
        tunnel: "T=sg\nF=bg" -> [w85]
        tunnel: [w84] -> w37 mode=indexing
        tunnel: [w83] -> w36 mode=indexing
        tunnel: [w82] -> w35 mode=indexing
        tunnel: [w81] -> w34 mode=indexing
        tunnel: [w79] -> w33 mode=indexing
        tunnel: [w67] -> w32 mode=indexing
        tunnel: [w68] -> w31 mode=indexing
        tunnel: [w78] -> w30 mode=indexing
        tunnel: [w77] -> w29 mode=indexing
        tunnel: [w76] -> w25 mode=indexing
        tunnel: [w75] -> w28 mode=indexing
        tunnel: [w74] -> w27
        tunnel: [w73] -> w24 mode=indexing
        tunnel: [w72] -> w23 mode=indexing
        tunnel: [w71] -> w22 mode=indexing
        tunnel: [w70] -> w21 mode=indexing
        tunnel: [w69] -> w20 mode=indexing
        tunnel: w19 -> [w66]
        i -> [w100]
        n8 = case shown="True" w85 {
          tunnel: w102 -> [w104 w110]
          tunnel: [w104 w106] -> w101
          tunnel: w92 -> [w103 w105]
          frame False {
            n9 = call <userlib>:"Voltage Update.vi"("Voltage Output"=w103) -> ()  [unwired: 8 in]
          }
          frame True {
            n10 = Unbundle By Name(w110) -> ("AO DC (V)"=w109:dbl[])
            n11 = Replace Array Subset(array=w109, new element=w105, index="\"channel\" side gate") -> (w107:dbl[])
            n12 = disable-structure shown="Disabled" {
              frame Disabled {
                (unwired) 3 ("index")
                n13 = Subtract(x=0.002) -> ()  [unwired: 1 in, 1 out]
              }
              frame Enabled {
              }
            }
            n14 = Bundle By Name(cluster=w110, "AO DC (V)"=w107) -> (w106:T1)
          }
        }
        n15 = Equal To 0?(x=w100) -> (x = 0?=w99:bool)
        n16 = stacked-sequence {
          tunnel: w101 -> [w112 _ _]
          tunnel: w92 -> [_ _ w131]
          tunnel: w99 -> [_ w114 w128]
          tunnel: [_ _ w172] -> w98
          tunnel: [_ _ w174] -> w97
          tunnel: [_ _ w173] -> w96
          tunnel: [_ _ w171] -> w95
          tunnel: [_ _ w170] -> w94
          tunnel: [_ _ w169] -> w93
          tunnel: [_ _ w165] -> w91
          tunnel: [_ _ w168] -> w90
          tunnel: [_ _ w167] -> w89
          tunnel: [_ _ w166] -> w88
          tunnel: [_ _ w153] -> w87
          tunnel: [_ _ w161] -> w86
          tunnel: [_ _ w158] -> w84
          tunnel: [_ _ w152] -> w83
          tunnel: [_ _ w151] -> w82
          tunnel: [_ _ w150] -> w81
          tunnel: [_ _ w149] -> w78
          tunnel: [_ _ w140] -> w77
          tunnel: [_ _ w148] -> w76
          tunnel: [_ _ w147] -> w75
          tunnel: [_ _ w141] -> w74
          tunnel: [_ _ w130] -> w73
          tunnel: [_ _ w139] -> w72
          tunnel: [_ _ w138] -> w71
          tunnel: [_ _ w137] -> w70
          tunnel: [_ _ w136] -> w69
          tunnel: w66 -> [_ _ _]
          frame #0 {
            n17 = disable-structure shown="Enabled" {
              frame Disabled {
                n18 = global read "Lock-in Globles Multiple Inputs and Outputs.vi" "OSC Configuration"() -> ()  [unwired: 1 in]
              }
              frame Enabled {
              }
            }
            n19 = call <userlib>:"FGV - Configuration - Output.vi"("Function"=enum16{"write", "read"}."write", "Channels: AO"=w112) -> ()  [unwired: 4 in, 2 out]
          }
          frame #1 {
            n20 = case shown="False" w114 {
              frame False {
                n21 = call <userlib>:"FGV - Signals - Input.vi"("Function"=enum16{"write", "read"}."read") -> ("input signal"=w117:waveform(dbl)[])  [unwired: 5 in, 1 out]
                n22 = Index Array(array=w117) -> (element=w116:waveform(dbl))  [unwired: 1 in]
                n23 = Unbundle By Name(w116) -> ("t0"=w115:timestamp)
                n24 = while {
                  shift-right: [w120] -> _
                  shift-left: w115 -> [w125]
                  stop <- w124 stop-if-true
                  n25 = call <userlib>:"FGV - Signals - Input.vi"("Function"=enum16{"write", "read"}."read") -> ("input signal"=w119:waveform(dbl)[])  [unwired: 5 in, 1 out]
                  n26 = Index Array(array=w119) -> (element=w122:waveform(dbl))  [unwired: 1 in]
                  n27 = Unbundle By Name(w122) -> ("t0"=w120:timestamp)
                  n28 = Not Equal?(x=w125, y=w120) -> (x != y?=w124:bool)
                  n29 = Wait (ms)(milliseconds to wait="wait between Vsgs") -> ()  [unwired: 1 out]
                }
              }
              frame True {
                n30 = Wait (ms)(milliseconds to wait="Initial wait") -> ()  [unwired: 1 out]
              }
            }
            n31 = disable-structure shown="Enabled" {
              frame Disabled {
                n32 = global read "Lock-in Globles Multiple Inputs and Outputs.vi" "timestamp"() -> ()  [unwired: 1 out]
              }
              frame Enabled {
              }
            }
          }
          frame #2 {
            # "Vsg"
            n33 = disable-structure shown="Enabled" {
              frame Disabled {
                n34 = global read "Lock-in Globles Multiple Inputs and Outputs.vi" "Results"() -> ()  [unwired: 1 out]
              }
              frame Enabled {
              }
            }
            n35 = call <userlib>:"FGV - Lockin Results.vi"("Function"=enum16{"write", "read"}."read") -> ("Input Signals"=w159:dbl[][])  [unwired: 5 in, 1 out]
            n36 = for {
              N: "# of lockins * #freq" -> [_]
              tunnel: w159 -> [w193]
              tunnel: [w191] -> w176 mode=indexing
              tunnel: [w190] -> w175 mode=indexing
              i -> [w192]
              # "extract x and y"
              n37 = Index Array(array=w193, index (row) #1=w192, index (col) #1=0 ("disabled index (col)"), index (row) #2=w192, index (col) #2=1 ("disabled index (col)")) -> (element #1=w191:dbl, element #2=w190:dbl)
            }
            n38 = Index Array(array=w175) -> (element #1=w173:dbl, element #2=w171:dbl, element #3=w169:dbl, element #4=w168:dbl, element #5=w166:dbl, element #6=w153:dbl, element #7=w152:dbl, element #8=w150:dbl, element #9=w140:dbl, element #10=w147:dbl)  [unwired: 10 in]
            n39 = Index Array(array=w176) -> (element #1=w174:dbl, element #2=w172:dbl, element #3=w170:dbl, element #4=w165:dbl, element #5=w167:dbl, element #6=w161:dbl, element #7=w158:dbl, element #8=w151:dbl, element #9=w149:dbl, element #10=w148:dbl, element #12=w130:dbl, element #13=w139:dbl, element #14=w138:dbl, element #15=w137:dbl, element #16=w136:dbl)  [unwired: 16 in, 1 out]
            n40 = call "Build XY Graph Vx2"("Reset"=w128, "Y Input"=w172, "X Input"=w131) -> ("XY Graph"=w178:cluster{"Y":dbl[], "Y":dbl[]}[])  [unwired: 2 in, 6 out]
            n41 = call "Build XY Graph Vx7"("Reset"=w128, "Y Input"=w165, "X Input"=w131) -> ("XY Graph"=w164:cluster{"Y":dbl[], "Y":dbl[]}[])  [unwired: 2 in, 6 out]
            n42 = call "Build XY Graph Vx6"("Reset"=w128, "Y Input"=w158, "X Input"=w131) -> ("XY Graph"=w157:cluster{"Y":dbl[], "Y":dbl[]}[])  [unwired: 2 in, 6 out]
            n43 = call "Build XY Graph Vx3"("Reset"=w128, "Y Input"=w170, "X Input"=w131) -> ("XY Graph"=w127:cluster{"Y":dbl[], "Y":dbl[]}[])  [unwired: 2 in, 6 out]
            n44 = call "Build XY Graph Vx4"("Reset"=w128, "Y Input"=w167, "X Input"=w131) -> ("XY Graph"=w163:cluster{"Y":dbl[], "Y":dbl[]}[])  [unwired: 2 in, 6 out]
            n45 = call "Build XY Graph Vx8"("Reset"=w128, "Y Input"=w151, "X Input"=w131) -> ("XY Graph"=w156:cluster{"Y":dbl[], "Y":dbl[]}[])  [unwired: 2 in, 6 out]
            n46 = call "Build XY Graph Vx9"("Reset"=w128, "Y Input"=w149, "X Input"=w131) -> ("XY Graph"=w155:cluster{"Y":dbl[], "Y":dbl[]}[])  [unwired: 2 in, 6 out]
            n47 = call "Build XY Graph Vx10"("Reset"=w128, "Y Input"=w148, "X Input"=w131) -> ("XY Graph"=w154:cluster{"Y":dbl[], "Y":dbl[]}[])  [unwired: 2 in, 6 out]
            n48 = call "Build XY Graph Vx5"("Reset"=w128, "Y Input"=w161, "X Input"=w131) -> ("XY Graph"=w162:cluster{"Y":dbl[], "Y":dbl[]}[])  [unwired: 2 in, 6 out]
            n49 = call "Build XY Graph Vx12"("Reset"=w128, "Y Input"=w139, "X Input"=w131) -> ("XY Graph"=w135:cluster{"Y":dbl[], "Y":dbl[]}[])  [unwired: 2 in, 6 out]
            n50 = call "Build XY Graph Vx15"("Reset"=w128, "Y Input"=w136, "X Input"=w131) -> ("XY Graph"=w132:cluster{"Y":dbl[], "Y":dbl[]}[])  [unwired: 2 in, 6 out]
            n51 = call "Build XY Graph Vx"("Reset"=w128, "Y Input"=w174, "X Input"=w131) -> ("XY Graph"=w179:cluster{"Y":dbl[], "Y":dbl[]}[])  [unwired: 2 in, 6 out]
            n52 = call "Build XY Graph Vx13"("Reset"=w128, "Y Input"=w138, "X Input"=w131) -> ("XY Graph"=w134:cluster{"Y":dbl[], "Y":dbl[]}[])  [unwired: 2 in, 6 out]
            n53 = call "Build XY Graph Vx14"("Reset"=w128, "Y Input"=w137, "X Input"=w131) -> ("XY Graph"=w133:cluster{"Y":dbl[], "Y":dbl[]}[])  [unwired: 2 in, 6 out]
            n54 = call "Build XY Graph Vx16"("Reset"=w128, "Y Input"=w130, "X Input"=w131) -> ("XY Graph"=w129:cluster{"Y":dbl[], "Y":dbl[]}[])  [unwired: 2 in, 6 out]
            n55 = Build Array (concatenate)(w179, w178, w127, w164, w163, w162, w157, w156, w155, w154, w129, w135, w134, w133, w132) -> (w146:cluster{"Y":dbl[], "Y":dbl[]}[])
            "Lockins" <- w146
            "Lockins 2" <- w146
            n56 = for {
              tunnel: w146 -> [w189]
              tunnel: [w183] -> w145 mode=indexing
              tunnel: "Current channels" -> [w182] mode=indexing
              tunnel: "Voltage channels" -> [w181] mode=indexing
              tunnel: [w180] -> w142 mode=indexing
              n57 = Index Array(array=w189, index #1=w182, index #2=w181) -> (element #1=w188:cluster{"Y":dbl[], "Y":dbl[]}, element #2=w187:cluster{"Y":dbl[], "Y":dbl[]})
              n58 = Unbundle(w187) -> ("Y"=w185:dbl[])  [unwired: 1 out]
              n59 = Unbundle(w188) -> ("Y"=w184:dbl[], "Y"=w186:dbl[])
              n60 = Divide(x=w186, y=w185) -> (x/y=w180:dbl[])
              n61 = Bundle("Y"=w184, w180) -> (w183:cluster{"Y":dbl[], dbl[]})  [unwired: 1 in]
            }
            "Lockins 3" <- w145
            n62 = Index Array(array=w142) -> (element=w141:dbl[])  [unwired: 2 in]
          }
        }
        n63 = global read "QDServGlobal.vi" "DR Field"() -> (w67:dbl)
        "Field" <- w67
        n64 = global read "QDServGlobal.vi" "DR Temperature"() -> (w68:dbl)
        "T (mK)" <- w68
        n65 = call <userlib>:"Read PPMS T and B.vi"() -> ()  [unwired: 3 in, 3 out]
        n66 = Get Date/Time In Seconds() -> (seconds since 1Jan1904=w80:timestamp)
        n67 = To Double Precision Float(number=w80) -> (double precision float=w79:dbl)
      }
      n68 = disable-structure shown="Disabled" {
        frame Disabled {
          n69 = local read "Channels: AO"() -> (w62:T1)
          n70 = local read "Vmin (start)"() -> (w63:dbl)
          n71 = local read "\"channel\" side gate"() -> (w65:i32)
          n72 = Unbundle By Name(w62) -> ("AO DC (V)"=w64:dbl[])
          n73 = Replace Array Subset(array=w64, new element=w63, index=w65) -> (w59:dbl[])
          n74 = Bundle By Name(cluster=w62, "AO DC (V)"=w59) -> (w60:T1)
          n75 = call <userlib>:"FGV - Configuration - Output.vi"("Function"=enum16{"write", "read"}."write", "Channels: AO"=w60) -> ()  [unwired: 4 in, 2 out]
        }
        frame Enabled {
        }
      }
      n76 = global read "ITX_Global.vi" "path"() -> (w58:path)
      n77 = Build Path(base path=w58, name or relative path="ITX folder") -> (appended path=w57:path)
      n78 = global read "ITX_Global.vi" "filename"() -> (w56:string)
      n79 = Build Cluster Array(w33, w26, w31, w32, w52, w51, w50, w49, w48, w47, w46, w45, w44, w43, w42, w41, w37, w36, w35, w34, w30, w29, w25, w28, w27, w24, w23, w22, w21, w20) -> (w55:cluster{"Waveform Graph":dbl[]}[])
      n80 = call <userlib>:"LV to ITX AutoPlot.vi"("filename"=w56, "path"=w57, "Notes"="Comments", "Data"=w55, "wavenames (.Vx, etc)"=string[] ["time", "Vsg", "T", "B", "X0", "Y0", "X1", "Y1", "X2", "Y2", "X3", "Y3", "X4", "Y4", "X5", "Y5", "X6", "Y6", "X7", "Y7", "X8", "Y8", "X9", "Y9", "Gcalc"]) -> ()  [unwired: 10 in, 1 out]
    }
  }
  n81 = disable-structure shown="Enabled" {
    frame Disabled {
      n82 = global read "Cryogeni Global 1.vi" "current RATE"() -> (w196:dbl)
      "ramp rate" <- w196
      n83 = Build Array(w196) -> ()  [unwired: 1 out]
    }
    frame Enabled {
    }
  }
